vi "DSF.Engine.Builder.Get Builder Status.vi"(11 "Builder in":refnum<class "DSF.Engine.Builder.lvclass">) -> (2 "Builder Status":refnum<class "Status.Builder.lvclass">, 3 "Builder out":refnum<class "DSF.Engine.Builder.lvclass">)   [LabVIEW 2017, in "DSF.Engine.lvlib" / "DSF.Engine.Builder.lvclass"]
uses:
  DSF.Engine.Builder.lvclass
  Status/Status.Builder.lvclass
  DSF.Engine.Builder.lvclass/DSF.Engine.Builder.ctl
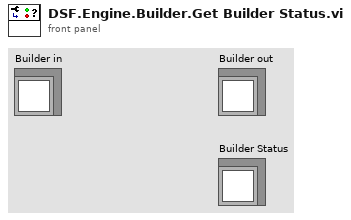
[diagram p1: front panel]
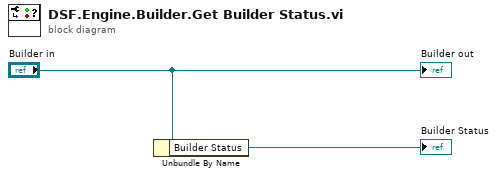
[diagram p0: block diagram]
diagram:
  n1 = Unbundle By Name("Builder in") -> ("Builder Status"=→"Builder Status":refnum<class "Status.Builder.lvclass">)
  "Builder out" <- "Builder in"
